vi "Build.vi"(0 "Export In":refnum<class "Export.lvclass">) -> (4 "Export Out":refnum<class "Export.lvclass">)   [LabVIEW 2017, in "CL_G3_VIComponentBuilder.lvlib" / "Export.lvclass"]
doc: "Creates the export artifacts, such as an executable, VI Package, DLL, etc."
uses:
  Export.lvclass
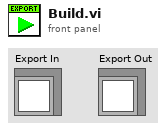
[diagram p1: front panel]
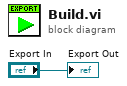
[diagram p0: block diagram]
diagram:
  "Export Out" <- "Export In"
